vi "PingTest.vi"(0 "IP/Address":string="127.0.0.1", 5 "PacketSize":i32=32, 7 "timeout":i32=100, 11 "Error in (no error)":errorcluster) -> (4 "Response":string, 6 "PingSuccess?":bool, 15 "Error out":errorcluster)   [LabVIEW 2017]
panel:
  out "Status":i32(ring) items=["Success"=0, "DestinationNetworkUnreachable"=11002, "DestinationHostUnreachable"=11003, "DestinationProhibited, DestinationProtocolUnreachable"=11004, "DestinationPortUnreachable"=11005, "NoResources"=11006, "BadOption"=11007, "HardwareError"=11008, "PacketTooBig"=11009, "TimedOut"=11010, "BadRoute"=11012, "TtlExpired"=11013, "TtlReassemblyTimeExceeded"=11014, "ParameterProblem"=11015, "SourceQuench"=11016, "BadDestination"=11018, "DestinationUnreachable"=11040, "TimeExceeded"=11041, "BadHeader"=11042, "UnrecognizedNextHeader"=11043, "IcmpError"=11044, "DestinationScopeMismatch"=11045, "Unknown"=-1]
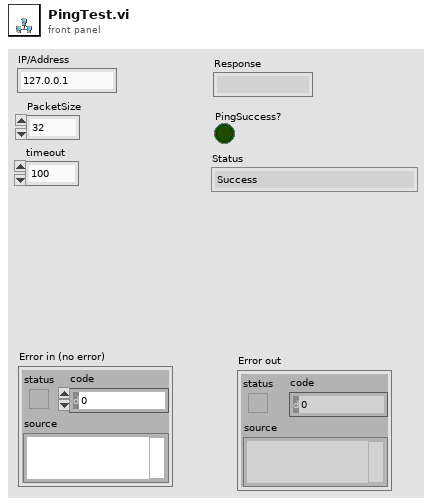
[diagram p1: front panel]
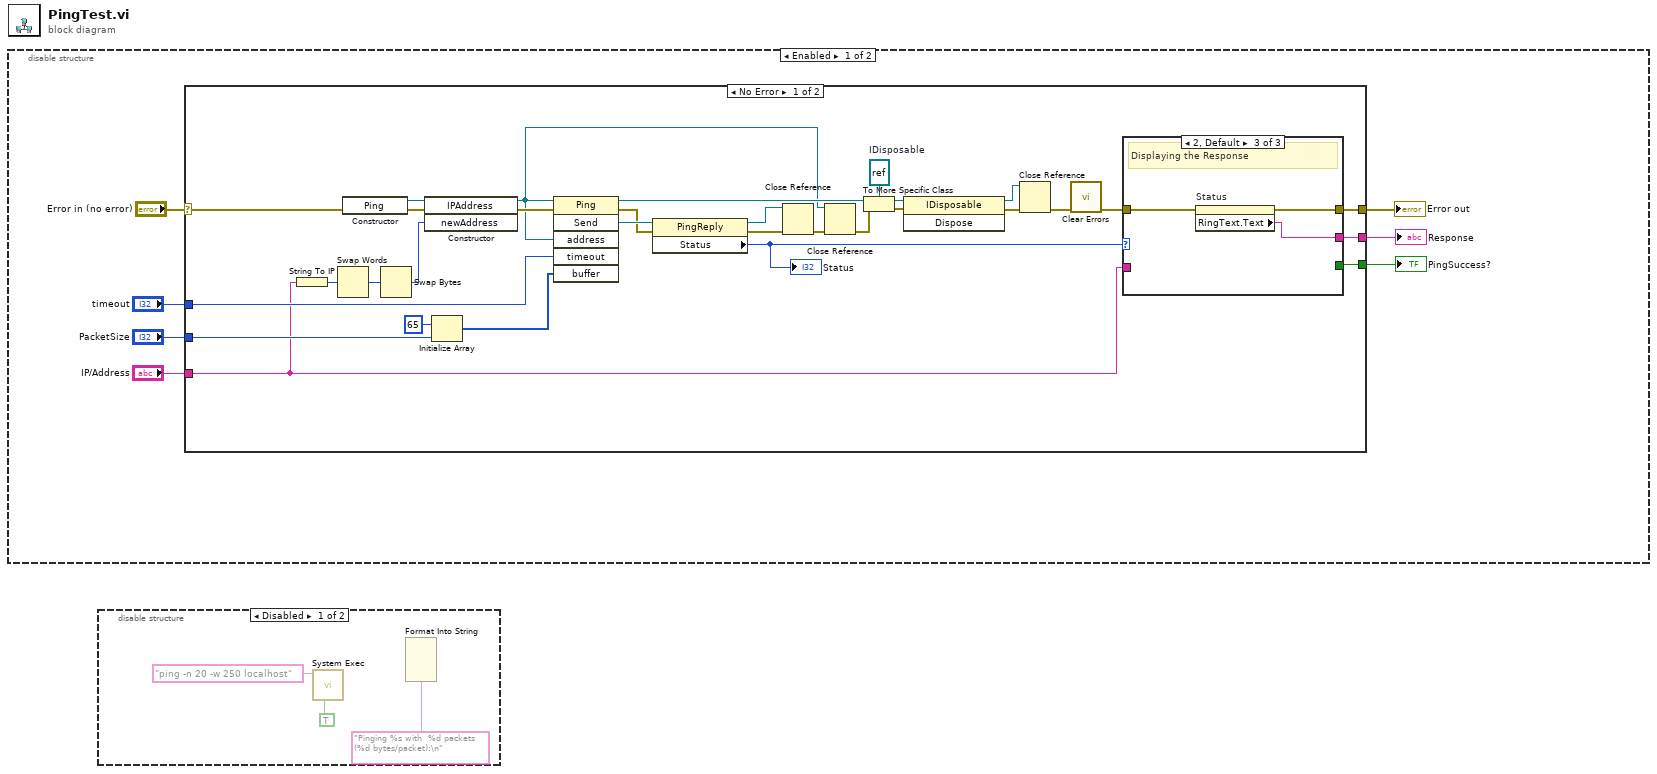
[diagram p0: block diagram]
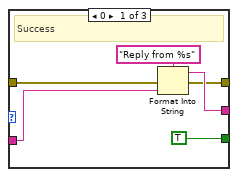
[diagram p3: hidden frame]
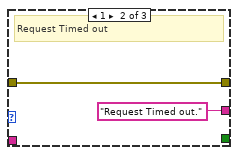
[diagram p4: hidden frame]
diagram:
  n1 = disable-structure shown="Enabled" {
    frame Enabled {
      n2 = case shown="No Error" "Error in (no error)" {
        selector: "Error in (no error)" -> [w8 w50]
        tunnel: "timeout" -> [w38 _]
        tunnel: "PacketSize" -> [w37 _]
        tunnel: "IP/Address" -> [w13 _]
        tunnel: [w12 _] -> w4
        tunnel: [w11 _] -> w3
        tunnel: [w9 w50] -> w2
        frame No Error {
          w27 = refnum<k24> refnum  # IDisposable
          n3 = String To IP(1:w13) -> (0:w31:u32)
          n4 = Swap Words(1:w31) -> (0:w29:u32)
          n5 = constructor class="Ping"(error in=w8) -> (reference out=w36:refnum<k24>, error out=w33:errorcluster)  [unwired: 2 in, 1 out]
          n6 = Swap Bytes(anything=w29) -> (byte swapped=w30:u32)
          n7 = constructor class="IPAddress"(error in=w33, "newAddress"=w30) -> (reference out=w23:refnum<k24>, error out=w32:errorcluster)  [unwired: 2 in, 2 out]
          n8 = Initialize Array(65, w37) -> (w35:i32[])
          n9 = invoke class="Ping" method="Send"(reference=w36, error in=w32, "address"=w23, "timeout"=w38, "buffer"=w35) -> (reference out=w28:refnum<k24>, error out=w15:errorcluster, "Send"=w16:refnum<k24>)  [unwired: 1 in, 3 out]
          n10 = property class="PingReply"(reference=w16, error in=w15) -> (reference out=w26:refnum<k24>, error out=w25:errorcluster, "Status"=w14:i32)
          "Status" <- w14
          n11 = Close Reference(reference=w26, error in (no error)=w25) -> (error out=w24:errorcluster)
          n12 = Close Reference(reference=w23, error in (no error)=w24) -> (error out=w22:errorcluster)
          n13 = To More Specific Class(target class=w27, reference=w28, error in=w22) -> (specific class reference=w21:refnum<k24>, error out=w20:errorcluster)
          n14 = invoke class="IDisposable" method="Dispose"(reference=w21, error in=w20) -> (reference out=w18:refnum<k24>, error out=w19:errorcluster)  [unwired: 1 in, 1 out]
          n15 = Close Reference(reference=w18, error in (no error)=w19) -> (error out=w17:errorcluster)
          n16 = call <vilib>:"Clear Errors.vi"("error in (no error)"=w17) -> ("error out"=w10:errorcluster)  [unwired: 5 in, 1 out]
          n17 = case shown="2, Default" w14 {
            tunnel: w13 -> [w44 _ _]
            tunnel: [w43 "Request Timed out." w47] -> w12
            tunnel: [TRUE _ _] -> w11
            tunnel: w10 -> [w41 w45 w49]
            tunnel: [w40 w45 w48] -> w9
            frame 0 {
              # "Success"
              n18 = Format Into String(format string="Reply from %s", error in=w41, w44) -> (resulting string=w43:string, error out=w40:errorcluster)  [unwired: 1 in]
            }
            frame 1 {
              # "Request Timed out"
            }
            frame 2, Default {
              # "Displaying the Response"
              n19 = property on="Status" class="Ring (strict)"(error in=w49) -> (error out=w48:errorcluster, "RingText.Text"=w47:string)  [unwired: 1 in, 1 out]
            }
          }
        }
        frame Error {
        }
      }
      "Error out" <- w2
      "Response" <- w4
      "PingSuccess?" <- w3
    }
    frame Disabled {
    }
  }
  n20 = disable-structure shown="Disabled" {
    frame Disabled {
      n21 = call <vilib>:"System Exec.vi"("run minimized? (F)"=TRUE, "command line"="ping -n 20 -w 250 localhost") -> ()  [unwired: 6 in, 4 out]
      n22 = Format Into String(format string="Pinging %s with  %d packets (%d bytes/packet):\n") -> ()  [unwired: 5 in, 2 out]
    }
    frame Enabled {
    }
  }
